vi "RSZVB Set IF Signal Port.vi"(8 "error in (no error)":errorcluster {"code" format="%.0x"}, 9 "Port Number (2)":i32=1, 10 "Channel (1)":i32=1, 11 "VISA resource name":refnum<visa-resource-name>) -> (0 "error out":errorcluster {"code" format="%.0x"}, 3 "VISA resource name out":refnum<visa-resource-name>)   [LabVIEW 2011]
doc: "This VI selects an analyzer port as receive port for the IF signal.\n\nNotes:\n\n(1) For mixer delay measurements and vector mixer measurements (options R&S ZVA-K5, R&S ZVA-K9, R&S ZVA-K10), the IF signal must be measured at port 2.\n\nRemote-control command(s):\n[SENSe<Ch>:]FREQuency:CONVersion:MIXer:IFPort <port_number>"
uses:
  _utility/RSZVB Global Data.vi
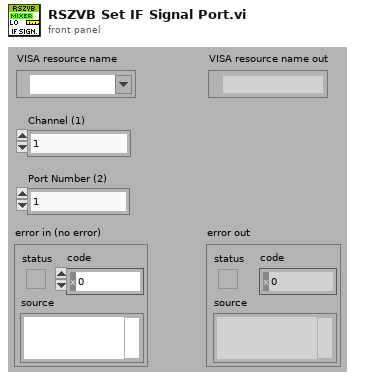
[diagram p1: front panel]
types:
  T1 = cluster{"Error Checking (T: On)":bool, "Installed Options":string[], "Data Valid?":bool, "Ports":i32, "Model":string[], "Option Checking (T: On)":bool}[]
  T2 = cluster{"Error Checking (T: On)":bool, "Installed Options":string[], "Data Valid?":bool, "Ports":i32, "Model":string[], "Option Checking (T: On)":bool}
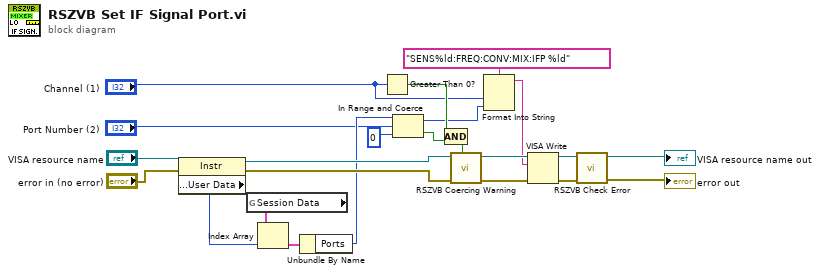
[diagram p0: block diagram]
diagram:
  n1 = property class="Instr"(reference="VISA resource name", error in="error in (no error)") -> (reference out=w13:refnum<visa-resource-name>, error out=w14:errorcluster, "General Settings:User Data"=w15:u32)
  n2 = global read "RSZVB Global Data.vi" "Session Data"() -> (w16:T1)
  n3 = Index Array(array=w16, index=w15) -> (element=w17:T2)
  n4 = Unbundle By Name(w17) -> ("Ports"=w12:i32)
  n5 = Greater Than 0?(x="Channel (1)") -> (x > 0?=w11:bool)
  n6 = In Range and Coerce(upper limit=w12, x="Port Number (2)", lower limit=0) -> (coerced(x)=w2:i32, In Range?=w5:bool)
  n7 = Compound Arithmetic op=AND(w11, w5) -> (w18:bool)
  n8 = call "RSZVB Coercing Warning.vi"("In Range?"=w18, "error in (no error)"=w14, "VISA session"=w13) -> ("error out"=w21:errorcluster, "dup VISA session"=w22:refnum<visa-resource-name>)  [unwired: 7 in]
  n9 = Format Into String(format string="SENS%ld:FREQ:CONV:MIX:IFP %ld", "Channel (1)", w2) -> (resulting string=w1:string)  [unwired: 2 in, 1 out]
  n10 = VISA Write(VISA resource name=w22, write buffer=w1, error in (no error)=w21) -> (VISA resource name out=w19:refnum<visa-resource-name>, error out=w20:errorcluster)  [unwired: 1 out]
  n11 = call "RSZVB Check Error.vi"("error in (no error)"=w20, "VISA session"=w19) -> ("error out"=→"error out":errorcluster, "dup VISA session"=→"VISA resource name out":refnum<visa-resource-name>)  [unwired: 8 in]
